vi "SE5082_Create_arb_waveform.vi"(5 "Reference phase (deg)":dbl, 7 "Reference frequency (MHz)":dbl=500.0, 8 "Variables":T1=[{"Value"=10.0, "Variable"="dummy", "Save with Image"=FALSE}, {"Value"=-0.0001, "Variable"="HI", "Save with Image"=FALSE}, {"Value"=-0.0002, "Variable"="LO", "Save with Image"=FALSE}, {"Value"=0.0, "Variable"="dummy1", "Save with Image"=FALSE}, {"Value"=0.0, "Variable"="dummy2", "Save with Image"=FALSE}, {"Value"=0.0, "Variable"="dummy3", "Save with Image"=FALSE}, {"Value"=0.0, "Variable"="tLEDuv", "Save with Image"=FALSE}, {"Value"=1000.0, "Variable"="tMOT0", "Save with Image"=FALSE}, {"Value"=20.0, "Variable"="tMOT1", "Save with Image"=FALSE}, {"Value"=40.0, "Variable"="tMOT2", "Save with Image"=FALSE}, {"Value"=50.0, "Variable"="tMOT3", "Save with Image"=FALSE}, {"Value"=13.0, "Variable"="tMOT3delayREP", "Save with Image"=FALSE}, {"Value"=0.05, "Variable"="tREP", "Save with Image"=FALSE}, {"Value"=0.75, "Variable"="dMOT0", "Save with Image"=FALSE}, {"Value"=1.75, "Variable"="dMOT1", "Save with Image"=FALSE}, {"Value"=1.75, "Variable"="dMOT2", "Save with Image"=FALSE}, {"Value"=0.0, "Variable"="dummy5", "Save with Image"=FALSE}, {"Value"=1.45, "Variable"="pMOT0", "Save with Image"=FALSE}, {"Value"=1.45, "Variable"="pMOT1", "Save with Image"=FALSE}, {"Value"=1.25, "Variable"="pMOT2", "Save with Image"=FALSE}, {"Value"=-1.0, "Variable"="dummy6", "Save with Image"=FALSE}, {"Value"=1.6, "Variable"="pRP0", "Save with Image"=FALSE}, {"Value"=1.6, "Variable"="pRP1", "Save with Image"=FALSE}, {"Value"=0.8, "Variable"="pRP2", "Save with Image"=FALSE}, {"Value"=0.0, "Variable"="MOTdummy0", "Save with Image"=FALSE}, {"Value"=-1.0, "Variable"="MOTdummy1", "Save with Image"=FALSE}, {"Value"=0.0, "Variable"="MOTdummy2", "Save with Image"=FALSE}, {"Value"=0.0, "Variable"="MOTdummy3", "Save with Image"=FALSE}, {"Value"=0.0, "Variable"="MOTdummy4", "Save with Image"=FALSE}, {"Value"=1.8, "Variable"="pCROSS0", "Save with Image"=FALSE}, {"Value"=1.29, "Variable"="pCROSS1", "Save with Image"=FALSE}, {"Value"=1.05, "Variable"="pCROSS2", "Save with Image"=FALSE}, {"Value"=0.75, "Variable"="pCROSS3", "Save with Image"=FALSE}, {"Value"=0.0, "Variable"="pCROSS4", "Save with Image"=FALSE}, {"Value"=5.0, "Variable"="pDIMPL0", "Save with Image"=FALSE}, {"Value"=4.4, "Variable"="pDIMPL1", "Save with Image"=FALSE}, {"Value"=3.65, "Variable"="pDIMPL2", "Save with Image"=FALSE}, {"Value"=3.55, "Variable"="pDIMPL3", "Save with Image"=FALSE}, {"Value"=3.45, "Variable"="pDIMPL4", "Save with Image"=FALSE}, {"Value"=1.8, "Variable"="pTightTrap", "Save with Image"=FALSE}, {"Value"=400.0, "Variable"="tHOLD", "Save with Image"=FALSE}, {"Value"=740.0, "Variable"="tEVAP1", "Save with Image"=FALSE}, {"Value"=2900.0, "Variable"="tEVAP2", "Save with Image"=FALSE}, {"Value"=590.0, "Variable"="tEVAP3", "Save with Image"=FALSE}, {"Value"=50.0, "Variable"="tEVAP4", "Save with Image"=FALSE}, {"Value"=50.0, "Variable"="tHOLDTight", "Save with Image"=FALSE}, {"Value"=0.0, "Variable"="ODTdummy1", "Save with Image"=FALSE}, {"Value"=0.0, "Variable"="ODTdummy2", "Save with Image"=FALSE}, {"Value"=0.0, "Variable"="ODTdummy3", "Save with Image"=FALSE}, {"Value"=0.0, "Variable"="ODTdummy4", "Save with Image"=FALSE}, {"Value"=0.0, "Variable"="ODTdummy5", "Save with Image"=FALSE}, {"Value"=3.59, "Variable"="dIMGx", "Save with Image"=FALSE}, {"Value"=3.59, "Variable"="dIMGx0", "Save with Image"=FALSE}, {"Value"=1.38, "Variable"="dIMGz", "Save with Image"=FALSE}, {"Value"=1.98, "Variable"="dEXCz", "Save with Image"=FALSE}, {"Value"=3.0, "Variable"="pABSx", "Save with Image"=FALSE}, {"Value"=1.35, "Variable"="pABSz", "Save with Image"=FALSE}, {"Value"=0.55, "Variable"="pEXCz", "Save with Image"=FALSE}, {"Value"=0.0, "Variable"="TOF", "Save with Image"=FALSE}, {"Value"=10.0, "Variable"="TOFatomFall", "Save with Image"=FALSE}, {"Value"=0.012, "Variable"="tEXP", "Save with Image"=FALSE}, {"Value"=0.2, "Variable"="tEXP2", "Save with Image"=FALSE}, {"Value"=0.082, "Variable"="tEXC", "Save with Image"=FALSE}, {"Value"=0.001, "Variable"="tWaitIoniz", "Save with Image"=FALSE}, {"Value"=0.065, "Variable"="tCAM", "Save with Image"=FALSE}, {"Value"=200.0, "Variable"="tCAMguppy", "Save with Image"=FALSE}, {"Value"=50.0, "Variable"="tCAMreadout", "Save with Image"=FALSE}, {"Value"=-0.002, "Variable"="tTrigDelay", "Save with Image"=FALSE}, {"Value"=0.0, "Variable"="tTrans", "Save with Image"=FALSE}, {"Value"=1.0, "Variable"="tEXCres", "Save with Image"=FALSE}, {"Value"=0.004, "Variable"="tPUMP", "Save with Image"=FALSE}, {"Value"=2.0, "Variable"="pBLUEswitch", "Save with Image"=FALSE}, {"Value"=2.0, "Variable"="pBLUEswitchEIT", "Save with Image"=FALSE}, {"Value"=3.5, "Variable"="dBLUE", "Save with Image"=FALSE}, {"Value"=3.5, "Variable"="dBLUE0", "Save with Image"=FALSE}, {"Value"=1.7, "Variable"="dBLUEdec", "Save with Image"=FALSE}, {"Value"=2.5, "Variable"="dBLUEdec0", "Save with Image"=FALSE}, {"Value"=3.2, "Variable"="dIMPnew", "Save with Image"=FALSE}, {"Value"=1.0, "Variable"="blueON1", "Save with Image"=FALSE}, {"Value"=0.0, "Variable"="blueON2", "Save with Image"=FALSE}, {"Value"=1.0, "Variable"="blueEXCON1", "Save with Image"=FALSE}, {"Value"=0.0, "Variable"="blueEXCON2", "Save with Image"=FALSE}, {"Value"=35.637858, "Variable"="dRydMW", "Save with Image"=FALSE}, {"Value"=16.0, "Variable"="pRydMW", "Save with Image"=FALSE}, {"Value"=50.0, "Variable"="MWduration", "Save with Image"=FALSE}, {"Value"=4.33, "Variable"="bmw0", "Save with Image"=FALSE}, {"Value"=0.02, "Variable"="bmw1", "Save with Image"=FALSE}, {"Value"=0.0, "Variable"="MWdummy1", "Save with Image"=FALSE}, {"Value"=0.0, "Variable"="MWdummy2", "Save with Image"=FALSE}, {"Value"=0.0, "Variable"="MWdummy3", "Save with Image"=FALSE}, {"Value"=4.3, "Variable"="foffset", "Save with Image"=FALSE}, {"Value"=8.64, "Variable"="fdx", "Save with Image"=FALSE}, {"Value"=-5.78, "Variable"="fdy", "Save with Image"=FALSE}, {"Value"=4.0, "Variable"="fdz", "Save with Image"=FALSE}, {"Value"=300.0, "Variable"="CH203", "Save with Image"=FALSE}, {"Value"=160.0, "Variable"="CH215", "Save with Image"=FALSE}, {"Value"=4.0, "Variable"="CH302", "Save with Image"=FALSE}, {"Value"=280.0, "Variable"="CH315", "Save with Image"=FALSE}, {"Value"=0.0, "Variable"="CH202", "Save with Image"=FALSE}, {"Value"=0.0, "Variable"="CH308", "Save with Image"=FALSE}, {"Value"=0.0, "Variable"="EFIELDdummy2", "Save with Image"=FALSE}, {"Value"=0.0, "Variable"="EFIELDdummy3", "Save with Image"=FALSE}, {"Value"=0.0, "Variable"="EFIELDdummy4", "Save with Image"=FALSE}, {"Value"=0.0, "Variable"="EFIELDdummy5", "Save with Image"=FALSE}, {"Value"=0.0, "Variable"="EFIELDdummy6", "Save with Image"=FALSE}, {"Value"=0.0, "Variable"="EFIELDdummy7", "Save with Image"=FALSE}, {"Value"=1.25, "Variable"="bMOT0", "Save with Image"=FALSE}, {"Value"=2.5, "Variable"="bMOT1", "Save with Image"=FALSE}, {"Value"=2.5, "Variable"="bMOT2", "Save with Image"=FALSE}, {"Value"=1.25, "Variable"="bMOT3", "Save with Image"=FALSE}, {"Value"=0.0, "Variable"="bCOMPx", "Save with Image"=FALSE}, {"Value"=1.35, "Variable"="bCOMPy", "Save with Image"=FALSE}, {"Value"=0.27, "Variable"="bCOMPz", "Save with Image"=FALSE}, {"Value"=0.7, "Variable"="bCOMPx1", "Save with Image"=FALSE}, {"Value"=1.1, "Variable"="bCOMPy1", "Save with Image"=FALSE}, {"Value"=0.5, "Variable"="bCOMPz1", "Save with Image"=FALSE}, {"Value"=4.35, "Variable"="bxfinal", "Save with Image"=FALSE}, {"Value"=0.0, "Variable"="byfinal", "Save with Image"=FALSE}, {"Value"=0.0, "Variable"="bzfinal", "Save with Image"=FALSE}, {"Value"=0.0, "Variable"="BFIELDdummy1", "Save with Image"=FALSE}, {"Value"=0.0, "Variable"="BFIELDdummy2", "Save with Image"=FALSE}, {"Value"=0.0, "Variable"="BFIELDdummy3", "Save with Image"=FALSE}, {"Value"=10.0, "Variable"="tCOILsettle", "Save with Image"=FALSE}, {"Value"=0.0, "Variable"="tRemove", "Save with Image"=FALSE}, {"Value"=3.6, "Variable"="pRemove", "Save with Image"=FALSE}, {"Value"=3.1, "Variable"="dF2CLEAN1x", "Save with Image"=FALSE}, {"Value"=20.0, "Variable"="tF2CLEAN1x", "Save with Image"=FALSE}, {"Value"=4.0, "Variable"="tF2CLEAN2x", "Save with Image"=FALSE}, {"Value"=0.0, "Variable"="tDelayDown", "Save with Image"=FALSE}, {"Value"=156.0, "Variable"="oDDSbluePro", "Save with Image"=FALSE}, {"Value"=-10.25, "Variable"="dDDSbluePro", "Save with Image"=FALSE}, {"Value"=50.0, "Variable"="tRampDDSbluePro", "Save with Image"=FALSE}, {"Value"=416.6261, "Variable"="oDDSred", "Save with Image"=FALSE}, {"Value"=-50.25, "Variable"="dDDSred", "Save with Image"=FALSE}, {"Value"=90.0, "Variable"="tRampDDSred", "Save with Image"=FALSE}, {"Value"=154.0, "Variable"="oDDSblueOld", "Save with Image"=FALSE}, {"Value"=10.0, "Variable"="dDDSblueOld", "Save with Image"=FALSE}, {"Value"=100.0, "Variable"="tRampDDSblueOld", "Save with Image"=FALSE}, {"Value"=1.0, "Variable"="mwON", "Save with Image"=FALSE}, {"Value"=9.4e-05, "Variable"="tRabi", "Save with Image"=FALSE}, {"Value"=9.4e-05, "Variable"="tRabi2", "Save with Image"=FALSE}, {"Value"=5e-05, "Variable"="tRamsey", "Save with Image"=FALSE}, {"Value"=0.0, "Variable"="tRamsey2", "Save with Image"=FALSE}, {"Value"=0.0, "Variable"="tDDSa", "Save with Image"=FALSE}, {"Value"=0.0, "Variable"="tDDSb", "Save with Image"=FALSE}, {"Value"=399.942, "Variable"="dDDSa", "Save with Image"=FALSE}, {"Value"=399.942, "Variable"="dDDSa2", "Save with Image"=FALSE}, {"Value"=0.2, "Variable"="pDDSa", "Save with Image"=FALSE}, {"Value"=1e-07, "Variable"="pDDSa2", "Save with Image"=FALSE}, {"Value"=0.0, "Variable"="phiDDSa", "Save with Image"=FALSE}, {"Value"=0.875, "Variable"="phiDDSa2", "Save with Image"=FALSE}, {"Value"=399.942, "Variable"="dDDSb", "Save with Image"=FALSE}, {"Value"=400.009, "Variable"="dDDSb2", "Save with Image"=FALSE}, {"Value"=0.25, "Variable"="pDDSb", "Save with Image"=FALSE}, {"Value"=1e-07, "Variable"="pDDSb2", "Save with Image"=FALSE}, {"Value"=0.25, "Variable"="phiDDSb", "Save with Image"=FALSE}, {"Value"=0.55, "Variable"="phiDDSb2", "Save with Image"=FALSE}, {"Value"=300.0, "Variable"="tDipole", "Save with Image"=FALSE}, {"Value"=0.7, "Variable"="bCOMPx2", "Save with Image"=FALSE}, {"Value"=0.8, "Variable"="bCOMPy2", "Save with Image"=FALSE}, {"Value"=0.6, "Variable"="bCOMPz2", "Save with Image"=FALSE}, {"Value"=20.0, "Variable"="dMOTRamp1", "Save with Image"=FALSE}, {"Value"=18.0, "Variable"="DMOTload", "Save with Image"=FALSE}, {"Value"=50.0, "Variable"="dMOTRamp2", "Save with Image"=FALSE}, {"Value"=272.0, "Variable"="DMOTimag", "Save with Image"=FALSE}, {"Value"=1000.0, "Variable"="oDDShyperfine", "Save with Image"=FALSE}, {"Value"=0.1, "Variable"="dDDShyperfine", "Save with Image"=FALSE}, {"Value"=0.0, "Variable"="tof", "Save with Image"=FALSE}, {"Value"=262.5, "Variable"="dOPump", "Save with Image"=FALSE}, {"Value"=4500.0, "Variable"="tRampOPump", "Save with Image"=FALSE}, {"Value"=10.0, "Variable"="tOPump", "Save with Image"=FALSE}, {"Value"=1.5, "Variable"="bCOMPx3", "Save with Image"=FALSE}, {"Value"=0.8, "Variable"="bCOMPy3", "Save with Image"=FALSE}, {"Value"=0.0, "Variable"="bCOMPz3", "Save with Image"=FALSE}, {"Value"=0.0, "Variable"="bCOMPx4", "Save with Image"=FALSE}, {"Value"=0.0, "Variable"="bCOMPy4", "Save with Image"=FALSE}, {"Value"=0.0, "Variable"="bCOMPz4", "Save with Image"=FALSE}, {"Value"=0.0, "Variable"="scan2photRes", "Save with Image"=FALSE}, {"Value"=0.0, "Variable"="tEXCsmallProbe", "Save with Image"=FALSE}, {"Value"=0.082, "Variable"="tEXCBlue", "Save with Image"=FALSE}, {"Value"=0.0015, "Variable"="tDownPump", "Save with Image"=FALSE}, {"Value"=98.75, "Variable"="RF1freq1", "Save with Image"=FALSE}, {"Value"=0.1, "Variable"="RF1freq2", "Save with Image"=FALSE}, {"Value"=98.75, "Variable"="dummya", "Save with Image"=FALSE}, {"Value"=0.011, "Variable"="dummyb", "Save with Image"=FALSE}] {"Value" format="%#.9g"}, 10 "waveform sequence":T3=[{"Waveform name"="Init X", "sequence duration (us)"=0.0, "Waveform"=[{"Segment number"=0, "frequency"="500", "phase"="0", "amplitude"="1", "duration"="dummyb", "envelope"=0}]}, {"Waveform name"="WAHUHA", "sequence duration (us)"=0.0, "Waveform"=[{"Segment number"=0, "frequency"="500", "phase"="0", "amplitude"="1", "duration"="0.01", "envelope"=0}, {"Segment number"=0, "frequency"="500", "phase"="0", "amplitude"="0", "duration"="0.01", "envelope"=0}, {"Segment number"=0, "frequency"="500", "phase"="90", "amplitude"="1", "duration"="0.01", "envelope"=0}, {"Segment number"=0, "frequency"="500", "phase"="90", "amplitude"="0", "duration"="0.02", "envelope"=0}, {"Segment number"=0, "frequency"="500", "phase"="270", "amplitude"="1", "duration"="0.01", "envelope"=0}, {"Segment number"=0, "frequency"="500", "phase"="270", "amplitude"="0", "duration"="0.01", "envelope"=0}, {"Segment number"=0, "frequency"="500", "phase"="180", "amplitude"="1", "duration"="0.01", "envelope"=0}, {"Segment number"=0, "frequency"="500", "phase"="180", "amplitude"="0", "duration"="0.01", "envelope"=0}]}, {"Waveform name"="Readout", "sequence duration (us)"=0.0, "Waveform"=[{"Segment number"=0, "frequency"="500", "phase"="0", "amplitude"="1", "duration"="0.03", "envelope"=0}]}] {"Waveform"."envelope" items=["Square", "Gaussian"]}, 11 "AWG sequence_variables":T2={"Sampling rate"=5000000000, "Channel"=1, "Sequence name"=0, "Save sequence"=FALSE, "Load waveform"=FALSE, "Waveform"=[{"Sequence on"=TRUE, "segment name"=0, "repeat"="1", "delay time"="0.001"}, {"Sequence on"=TRUE, "segment name"=1, "repeat"="1", "delay time"="0.005"}, {"Sequence on"=TRUE, "segment name"=2, "repeat"="1", "delay time"="0"}]} {"Sequence name" items=["Init X", "WAHUHA", "Readout X", "New waveform..."]; "Channel" format="%.0p"; "Sampling rate" format="%.0p"; "Waveform"."segment name" items=["Init X", "WAHUHA", "Readout X"]}) -> (1 "ref amplitude":dbl[](array[numeric]), 2 "y":dbl[](array[numeric]), 3 "x":dbl[](array[numeric]))   [LabVIEW 2017]
uses:
  waveform_variables_new.ctl
  sequence_variables.ctl
  Software/Rydberg_Control/TypeDefinition/variables.ctl
panel:
  out "size ref (new)":i32=4736
  out "size ref":i32=4736
  out "size y (new)":i32=4736
  out "segment name":string[](array[string])
  out "Step size (ns)":dbl=0.2
  out "XY Graph all":cluster{dbl[], "y":dbl[]}[](graph)
  out "XY Graph":cluster{dbl[], "y":dbl[]}[](graph)
  out "all duration":i32[](array[numeric])=[55, 50, 50, 50, 100, 50, 50, 50, 50, 50, 50, 50, 100, 50, 50, 50, 50, 50, 50, 50, 100, 50, 50, 50, 50, 50, 50, 50, 100, 50, 50, 50, 50, 50, 50, 50, 100, 50, 50, 50, 50, 50, 50, 50, 100, 50, 50, 50, 50, 50, 50, 50, 100, 50, 50, 50, 50, 50, 50, 50, 100, 50, 50, 50, 50, 50, 50, 50, 100, 50, 50, 50, 50, 50, 50, 50, 100, 50, 50, 50, 50, 150, 30]
  out "all frequency":dbl[](array[numeric])=[500.0, 500.0, 500.0, 500.0, 500.0, 500.0, 500.0, 500.0, 500.0, 500.0, 500.0, 500.0, 500.0, 500.0, 500.0, 500.0, 500.0, 500.0, 500.0, 500.0, 500.0, 500.0, 500.0, 500.0, 500.0, 500.0, 500.0, 500.0, 500.0, 500.0, 500.0, 500.0, 500.0, 500.0, 500.0, 500.0, 500.0, 500.0, 500.0, 500.0, 500.0, 500.0, 500.0, 500.0, 500.0, 500.0, 500.0, 500.0, 500.0, 500.0, 500.0, 500.0, 500.0, 500.0, 500.0, 500.0, 500.0, 500.0, 500.0, 500.0, 500.0, 500.0, 500.0, 500.0, 500.0, 500.0, 500.0, 500.0, 500.0, 500.0, 500.0, 500.0, 500.0, 500.0, 500.0, 500.0, 500.0, 500.0, 500.0, 500.0, 500.0, 500.0, 500.0]
  out "all phase":dbl[](array[numeric])=[0.0, 0.0, 0.0, 90.0, 90.0, 270.0, 270.0, 180.0, 180.0, 0.0, 0.0, 90.0, 90.0, 270.0, 270.0, 180.0, 180.0, 0.0, 0.0, 90.0, 90.0, 270.0, 270.0, 180.0, 180.0, 0.0, 0.0, 90.0, 90.0, 270.0, 270.0, 180.0, 180.0, 0.0, 0.0, 90.0, 90.0, 270.0, 270.0, 180.0, 180.0, 0.0, 0.0, 90.0, 90.0, 270.0, 270.0, 180.0, 180.0, 0.0, 0.0, 90.0, 90.0, 270.0, 270.0, 180.0, 180.0, 0.0, 0.0, 90.0, 90.0, 270.0, 270.0, 180.0, 180.0, 0.0, 0.0, 90.0, 90.0, 270.0, 270.0, 180.0, 180.0, 0.0, 0.0, 90.0, 90.0, 270.0, 270.0, 180.0, 180.0, 0.0, 0.0]
  out "all amplitude":dbl[](array[numeric])=[1.0, 1.0, 0.0, 1.0, 0.0, 1.0, 0.0, 1.0, 0.0, 1.0, 0.0, 1.0, 0.0, 1.0, 0.0, 1.0, 0.0, 1.0, 0.0, 1.0, 0.0, 1.0, 0.0, 1.0, 0.0, 1.0, 0.0, 1.0, 0.0, 1.0, 0.0, 1.0, 0.0, 1.0, 0.0, 1.0, 0.0, 1.0, 0.0, 1.0, 0.0, 1.0, 0.0, 1.0, 0.0, 1.0, 0.0, 1.0, 0.0, 1.0, 0.0, 1.0, 0.0, 1.0, 0.0, 1.0, 0.0, 1.0, 0.0, 1.0, 0.0, 1.0, 0.0, 1.0, 0.0, 1.0, 0.0, 1.0, 0.0, 1.0, 0.0, 1.0, 0.0, 1.0, 0.0, 1.0, 0.0, 1.0, 0.0, 1.0, 0.0, 1.0, 0.0]
  out "time for waveform":dbl[](array[numeric])=[0.0, 1.1e-08, 2.1e-08, 3.1e-08, 4.1e-08, 6.1e-08, 7.1e-08, 8.1e-08, 9.1e-08, 1.01e-07, 1.11e-07, 1.21e-07, 1.31e-07, 1.51e-07, 1.61e-07, 1.71e-07, 1.81e-07, 1.91e-07, 2.01e-07, 2.11e-07, 2.21e-07, 2.41e-07, 2.51e-07, 2.61e-07, 2.71e-07, 2.81e-07, 2.91e-07, 3.01e-07, 3.11e-07, 3.31e-07, 3.41e-07, 3.51e-07, 3.61e-07, 3.71e-07, 3.81e-07, 3.91e-07, 4.01e-07, 4.21e-07, 4.31e-07, 4.41e-07, 4.51e-07, 4.61e-07, 4.71e-07, 4.81e-07, 4.91e-07, 5.11e-07, 5.21e-07, 5.31e-07, 5.41e-07, 5.51e-07, 5.61e-07, 5.71e-07, 5.81e-07, 6.01e-07, 6.11e-07, 6.21e-07, 6.31e-07, 6.41e-07, 6.51e-07, 6.61e-07, 6.71e-07, 6.91e-07, 7.01e-07, 7.11e-07, 7.21e-07, 7.31e-07, 7.41e-07, 7.51e-07, 7.61e-07, 7.81e-07, 7.91e-07, 8.01e-07, 8.11e-07, 8.21e-07, 8.31e-07, 8.41e-07, 8.51e-07, 8.71e-07, 8.81e-07, 8.91e-07, 9.01e-07, 9.11e-07, 9.41e-07]
  out "input amplitude":dbl[](array[numeric])=[1.0, 1.0, 0.0, 1.0, 0.0, 1.0, 0.0, 1.0, 0.0, 1.0, 0.0, 1.0, 0.0, 1.0, 0.0, 1.0, 0.0, 1.0, 0.0, 1.0, 0.0, 1.0, 0.0, 1.0, 0.0, 1.0, 0.0, 1.0, 0.0, 1.0, 0.0, 1.0, 0.0, 1.0, 0.0, 1.0, 0.0, 1.0, 0.0, 1.0, 0.0, 1.0, 0.0, 1.0, 0.0, 1.0, 0.0, 1.0, 0.0, 1.0, 0.0, 1.0, 0.0, 1.0, 0.0, 1.0, 0.0, 1.0, 0.0, 1.0, 0.0, 1.0, 0.0, 1.0, 0.0, 1.0, 0.0, 1.0, 0.0, 1.0, 0.0, 1.0, 0.0, 1.0, 0.0, 1.0, 0.0, 1.0, 0.0, 1.0, 0.0, 1.0]
  out "input phase":dbl[](array[numeric])=[0.0, 0.0, 0.0, 90.0, 90.0, 270.0, 270.0, 180.0, 180.0, 0.0, 0.0, 90.0, 90.0, 270.0, 270.0, 180.0, 180.0, 0.0, 0.0, 90.0, 90.0, 270.0, 270.0, 180.0, 180.0, 0.0, 0.0, 90.0, 90.0, 270.0, 270.0, 180.0, 180.0, 0.0, 0.0, 90.0, 90.0, 270.0, 270.0, 180.0, 180.0, 0.0, 0.0, 90.0, 90.0, 270.0, 270.0, 180.0, 180.0, 0.0, 0.0, 90.0, 90.0, 270.0, 270.0, 180.0, 180.0, 0.0, 0.0, 90.0, 90.0, 270.0, 270.0, 180.0, 180.0, 0.0, 0.0, 90.0, 90.0, 270.0, 270.0, 180.0, 180.0, 0.0, 0.0, 90.0, 90.0, 270.0, 270.0, 180.0, 180.0, 0.0]
  out "input frequency":dbl[](array[numeric])=[500.0, 500.0, 500.0, 500.0, 500.0, 500.0, 500.0, 500.0, 500.0, 500.0, 500.0, 500.0, 500.0, 500.0, 500.0, 500.0, 500.0, 500.0, 500.0, 500.0, 500.0, 500.0, 500.0, 500.0, 500.0, 500.0, 500.0, 500.0, 500.0, 500.0, 500.0, 500.0, 500.0, 500.0, 500.0, 500.0, 500.0, 500.0, 500.0, 500.0, 500.0, 500.0, 500.0, 500.0, 500.0, 500.0, 500.0, 500.0, 500.0, 500.0, 500.0, 500.0, 500.0, 500.0, 500.0, 500.0, 500.0, 500.0, 500.0, 500.0, 500.0, 500.0, 500.0, 500.0, 500.0, 500.0, 500.0, 500.0, 500.0, 500.0, 500.0, 500.0, 500.0, 500.0, 500.0, 500.0, 500.0, 500.0, 500.0, 500.0, 500.0, 500.0]
  out "input duration":i32[](array[numeric])=[55, 50, 50, 50, 100, 50, 50, 50, 50, 50, 50, 50, 100, 50, 50, 50, 50, 50, 50, 50, 100, 50, 50, 50, 50, 50, 50, 50, 100, 50, 50, 50, 50, 50, 50, 50, 100, 50, 50, 50, 50, 50, 50, 50, 100, 50, 50, 50, 50, 50, 50, 50, 100, 50, 50, 50, 50, 50, 50, 50, 100, 50, 50, 50, 50, 50, 50, 50, 100, 50, 50, 50, 50, 50, 50, 50, 100, 50, 50, 50, 50, 150]
  out "repeat":i32[](array[numeric])=[1, 10, 1]
  out "segment number":u16[](array[numeric])=[0, 1, 2]
  out "sequence on":bool[](array[boolean])=[TRUE, TRUE, TRUE]
  in  "Plot waveform":bool
  in  "Waveform name":u16(ring) items=["Init X", "WAHUHA", "Readout X", "New waveform..."]
  in  "Save waveform":bool
  out "size y":i32=4736
  out "total samples":i32=4736
  out "samples to add":i32=30
  out "segment init phase":dbl[](array[numeric])=[0.0, 179.99999999999977, 180.00000000000045, 180.0, 180.00000000000182, 179.99999999999818, 180.0, 180.0, 180.0, 180.0, 180.0, 180.00000000000364, 180.0, 180.0, 179.99999999999636, 180.0, 180.0, 180.0, 180.0, 180.0, 180.0, 180.00000000000728, 180.00000000000728, 180.00000000000728, 179.99999999999272, 179.99999999999272, 179.99999999999272, 180.0, 180.0, 180.0, 180.00000000000728, 180.0, 180.00000000000728, 180.0, 180.0, 180.0, 180.0, 180.00000000001455, 180.0, 180.0, 180.0, 180.0, 180.0, 180.00000000001455, 180.0, 180.0, 180.00000000001455, 180.0, 180.0, 180.00000000001455, 180.0, 180.00000000001455, 180.0, 180.0000000000291, 180.0, 179.99999999998545, 179.99999999998545, 180.0, 179.99999999998545, 180.0, 180.00000000001455, 180.0, 180.00000000001455, 179.99999999998545, 180.0, 180.0, 180.0, 179.9999999999709, 180.0, 180.0, 180.0000000000291, 180.0, 180.0, 180.0, 180.0, 180.0, 180.0000000000291, 180.0, 180.0, 180.0, 180.0000000000291, 180.0000000000291, 180.0]
  out "ref phase(deg)":dbl[](array[numeric])
  out "Reference phase":cluster{"x":dbl[], "y":dbl[]}(graph)
  out "Plot X":dbl[](graph)
  out "Plot Y":dbl[](graph)
  out "y (original)":dbl[](array[numeric])
  out "Sampling rate":i64=5000000000
  out "Reference amplitude":cluster{"x":dbl[], "y":dbl[]}(graph)
  # "Max 5 GSa/s"
  # "1 or 2"
  # "ON?"
  # "segment name"
  # "repeat"
  # "delay time (us)"
  # "No."
  # "freq (MHz)"
  # "phase  (deg)"
  # "amplitude (0-1)"
  # "duration (us)"
  # "envelope"
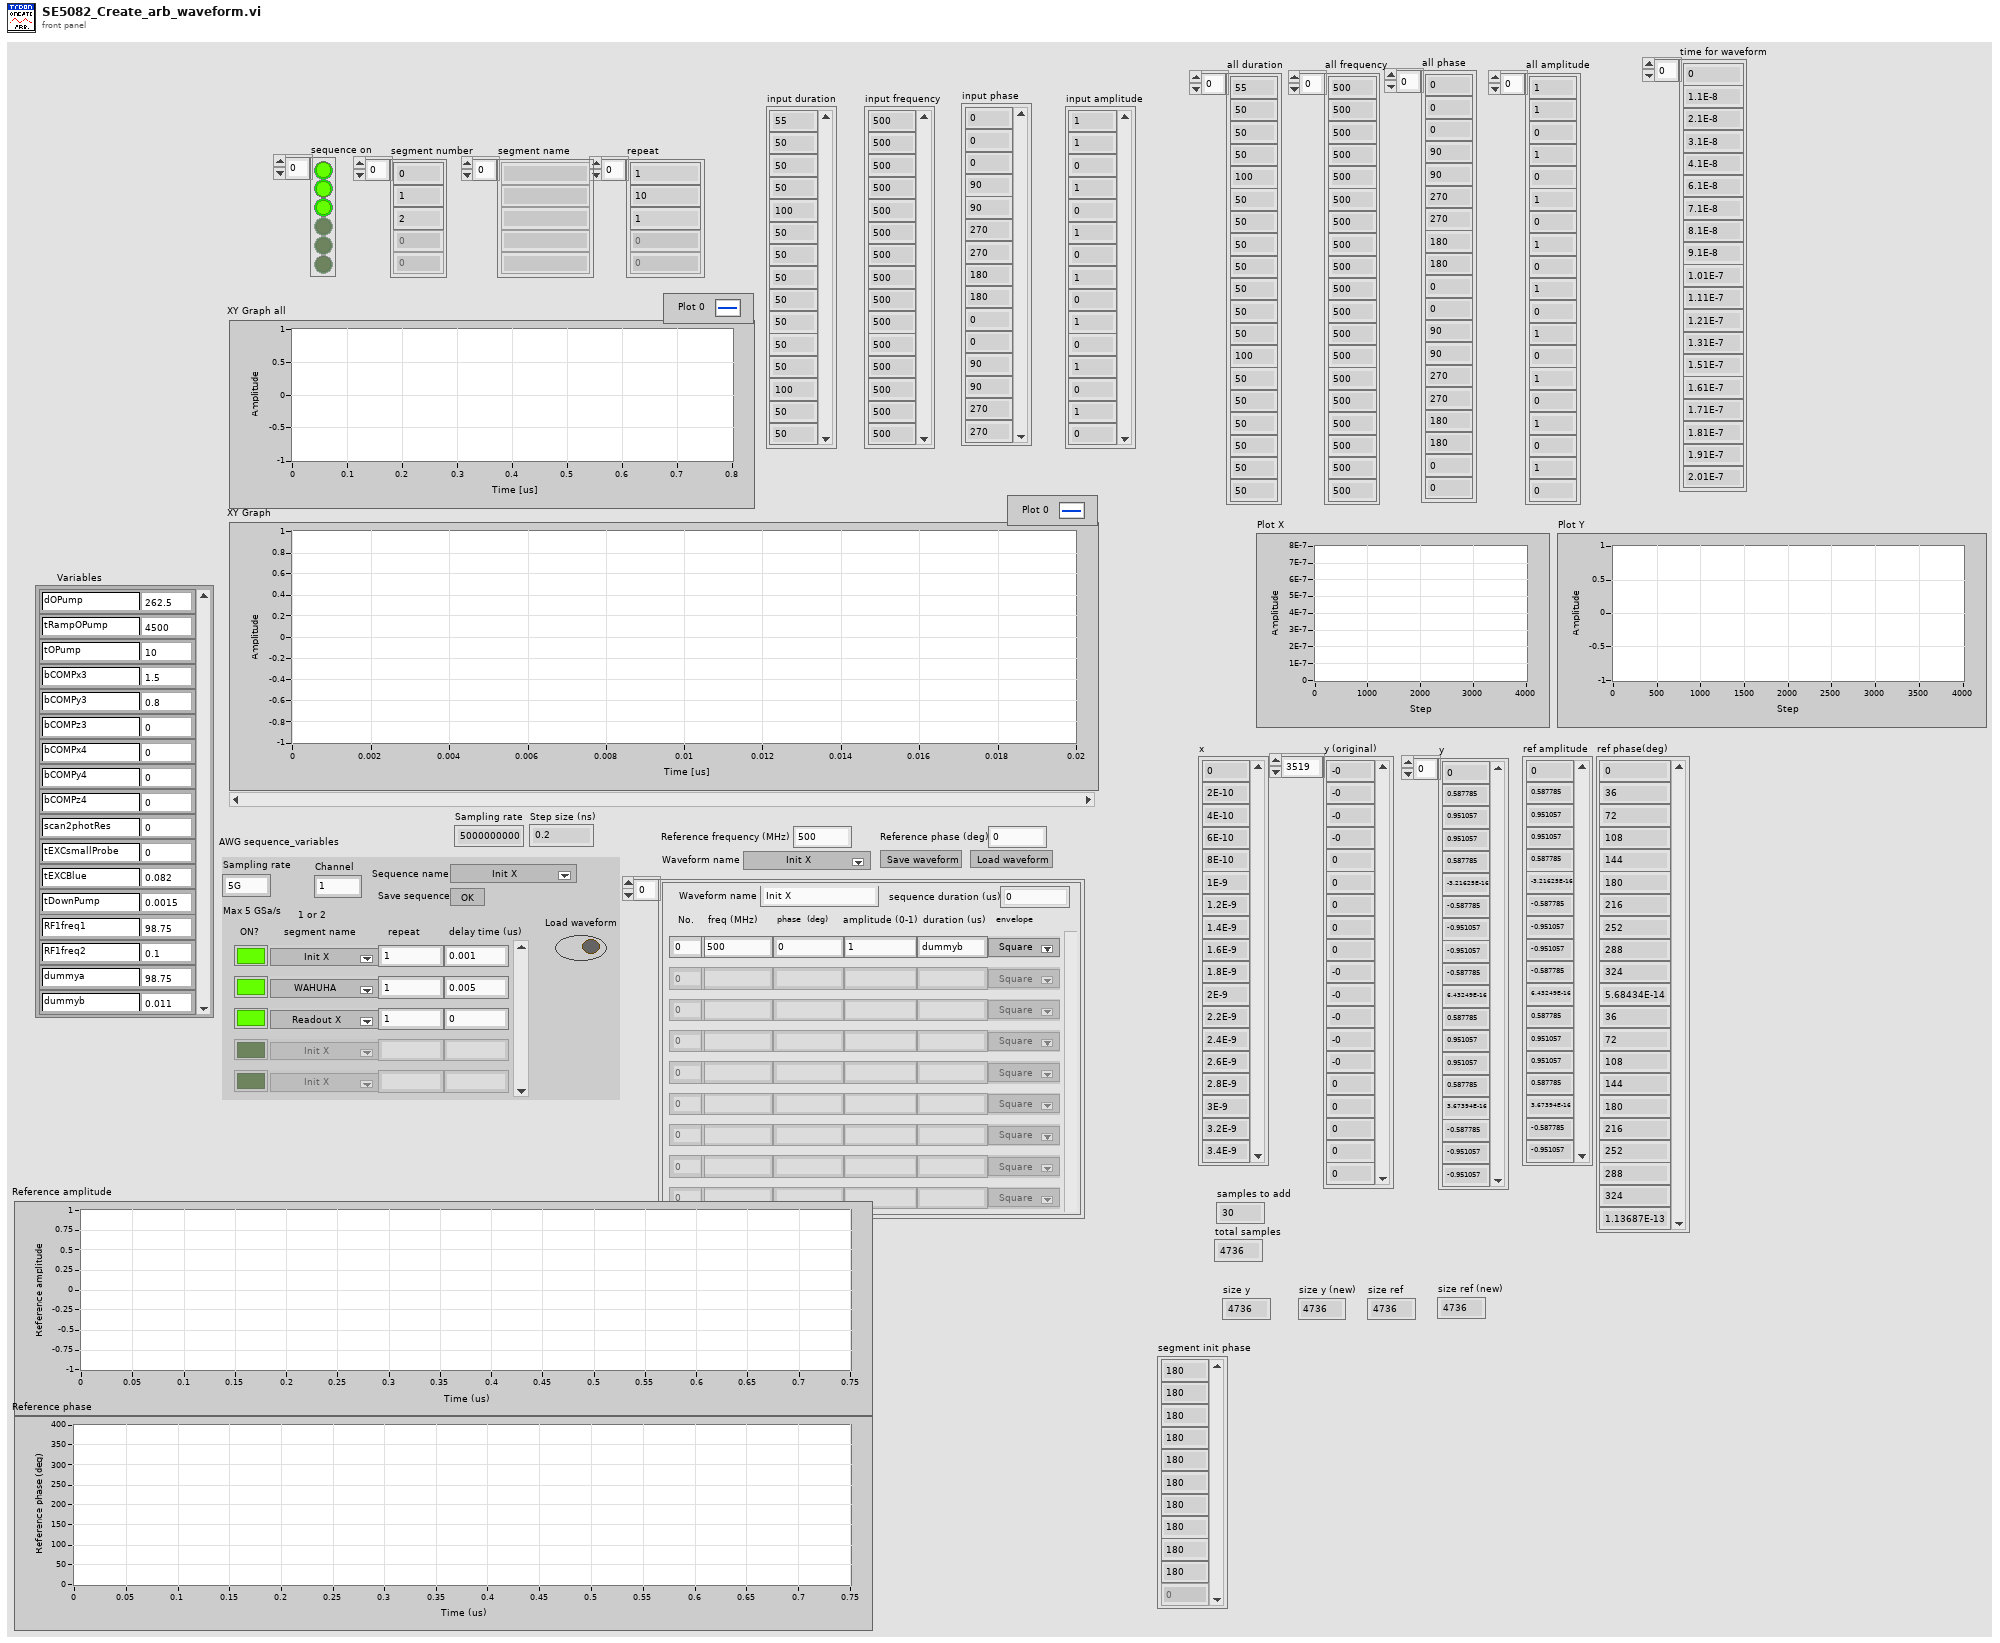
[diagram p1: front panel]
types:
  T1 = typedef "variables.ctl" = cluster{"Value":dbl, "Variable":string, "Save with Image":bool}[]
  T2 = typedef "sequence_variables.ctl" = cluster{"Sampling rate":i64, "Channel":i8, "Sequence name":u16, "Save sequence":bool, "Load waveform":bool, "Waveform":cluster{"Sequence on":bool, "segment name":u16, "repeat":string, "delay time":string}[]}
  T3 = typedef "waveform_variables_new.ctl" = cluster{"Waveform name":string, "sequence duration (us)":dbl, "Waveform":cluster{"Segment number":i32, "frequency":string, "phase":string, "amplitude":string, "duration":string, "envelope":u16}[]}[]
  T4 = cluster{"Sequence on":bool, "segment name":u16, "repeat":string, "delay time":string}[]
  T5 = cluster{"Waveform name":string, "sequence duration (us)":dbl, "Waveform":cluster{"Segment number":i32, "frequency":string, "phase":string, "amplitude":string, "duration":string, "envelope":u16}[]}
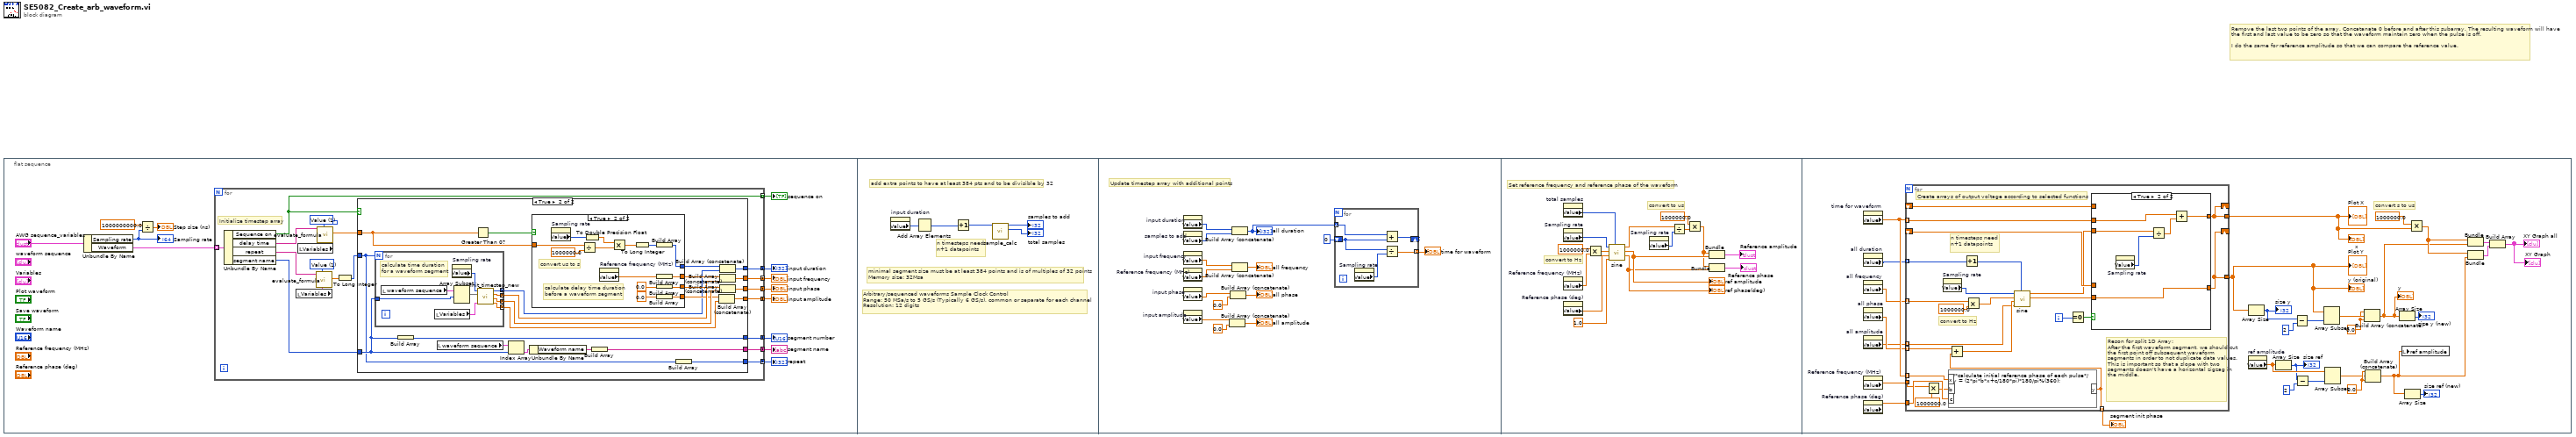
[diagram p0: block diagram]
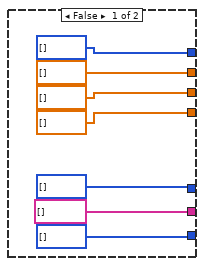
[diagram p2: hidden frame]
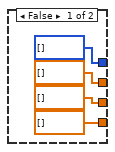
[diagram p3: hidden frame]
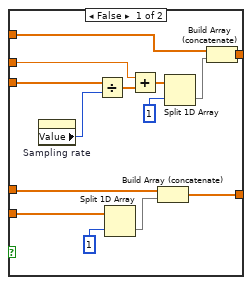
[diagram p4: hidden frame]
diagram:
  # "Remove the last two points of the array. Concatanate 0 before and after this subarray. The resulting waveform will have the first and last value to be zero so that the waveform maintain zero when the pulse is off.\n\nI do the same for reference amplitude so that we can compare the reference value."
  n1 = flat-sequence {
    frame #0 {
      n2 = Unbundle By Name("AWG sequence_variables") -> ("Sampling rate"=w10:i64, "Waveform"=w5:T4)
      "Sampling rate" <- w10
      n3 = Divide(x=1000000000.0, y=w10) -> (x/y=→"Step size (ns)":dbl)
      n4 = for {
        tunnel: w5 -> [w32] mode=indexing
        tunnel: [w26] -> w3 mode=indexing
        tunnel: [w18] -> w4 mode=concatenating
        tunnel: [w24] -> w9 mode=concatenating
        tunnel: [w23] -> w6 mode=concatenating
        tunnel: [w22] -> w7 mode=concatenating
        tunnel: [w21] -> w8 mode=concatenating
        tunnel: [w20] -> w12 mode=concatenating
        tunnel: [w19] -> w13 mode=concatenating
        w14 = u16 1 items=["Time in counts", "Value"] ("Time or Value")
        w30 = u16 1 items=["Time in counts", "Value"] ("Time or Value")
        # "Initialize timestep array"
        n5 = Unbundle By Name(w32) -> ("Sequence on"=w26:bool, "delay time"=w27:string, "repeat"=w16:string, "segment name"=w15:u16)
        n6 = local read "Variables"() -> (w31:T1)
        n7 = local read "Variables"() -> (w28:T1)
        n8 = call "evaluate_formula.vi"("Variable array"=w31, "Time or Value"=w30, "Formula"=w16) -> ("Output"=w29:dbl)  [unwired: 7 in, 1 out]
        n9 = call "evaluate_formula.vi"("Variable array"=w28, "Time or Value"=w14, "Formula"=w27) -> ("Output"=w17:dbl)  [unwired: 7 in, 1 out]
        n10 = To Long Integer(number=w29) -> (32bit integer=w25:i32)
        n11 = case shown="True" w26 {
          tunnel: w15 -> [_ w56]
          tunnel: w25 -> [_ w55]
          tunnel: [i32[] [] ("segment duration (int)") w51] -> w24
          tunnel: [dbl[] [] ("segment frequency") w49] -> w23
          tunnel: [dbl[] [] ("segment phase") w48] -> w22
          tunnel: [dbl[] [] ("segment amplitude") w47] -> w21
          tunnel: [string[] [] w58] -> w20
          tunnel: [u16[] [] w57] -> w19
          tunnel: [i32[] [] w54] -> w18
          tunnel: w17 -> [_ w52]
          frame False {
          }
          frame True {
            n12 = for {
              N: w55 -> [_]
              tunnel: w56 -> [w84]
              tunnel: [w83] -> w40 mode=concatenating
              tunnel: [w82] -> w46 mode=concatenating
              tunnel: [w81] -> w45 mode=concatenating
              tunnel: [w80] -> w44 mode=concatenating
              # "calculate time duration\nfor a waveform segment"
              n13 = local read "waveform sequence"() -> (w87:T3)
              n14 = local read "Variables"() -> (w85:T1)
              n15 = property on="Sampling rate" class="DigNum (strict)"() -> ("Value"=w86:i64)  [unwired: 2 in, 2 out]
              n16 = Array Subset(array=w87, index=w84) -> (w88:T3)  [unwired: 1 in]
              n17 = call "Init_timestep_new.vi"("Variables"=w85, "waveform sequence"=w88, "Sampling rate"=w86) -> ("segment amplitude"=w80:dbl[], "segment phase"=w81:dbl[], "segment frequency"=w82:dbl[], "segment duration (int)"=w83:i32[])  [unwired: 5 in]
            }
            n18 = Build Array(w56) -> (w57:u16[])
            n19 = local read "waveform sequence"() -> (w61:T3)
            n20 = Greater Than 0?(x=w52) -> (x > 0?=w53:bool)
            n21 = Index Array(array=w61, index=w56) -> (element=w60:T5)
            n22 = Unbundle By Name(w60) -> ("Waveform name"=w59:string)
            n23 = case shown="True" w53 {
              tunnel: w52 -> [_ w76]
              tunnel: [i32[] [] w74] -> w50
              tunnel: [dbl[] [] w70] -> w43
              tunnel: [dbl[] [] w69] -> w42
              tunnel: [dbl[] [] w68] -> w41
              frame False {
              }
              frame True {
                # "calculate delay time duration\nbefore a waveform segment"
                # "convert us to s"
                n24 = property on="Sampling rate" class="DigNum (strict)"() -> ("Value"=w67:i64)  [unwired: 2 in, 2 out]
                n25 = Divide(x=w76, y=1000000.0) -> (x/y=w78:dbl)
                n26 = To Double Precision Float(number=w67) -> (double precision float=w66:dbl)
                n27 = property on="Reference frequency (MHz)" class="DigNum (strict)"() -> ("Value"=w73:dbl)  [unwired: 2 in, 2 out]
                n28 = Multiply(x=w66, y=w78) -> (x*y=w79:dbl)
                n29 = To Long Integer(number=w79) -> (32bit integer=w75:i32)
                n30 = Build Array(w75) -> (w74:i32[])
                n31 = Build Array(w73) -> (w70:dbl[])
                n32 = Build Array(0.0 ("element")) -> (w69:dbl[])
                n33 = Build Array(0.0 ("element")) -> (w68:dbl[])
              }
            }
            n34 = Build Array(w59) -> (w58:string[])
            n35 = Build Array(w55) -> (w54:i32[])
            n36 = Build Array (concatenate)(w41, w44) -> (w47:dbl[])
            n37 = Build Array (concatenate)(w50, w40) -> (w51:i32[])
            n38 = Build Array (concatenate)(w43, w46) -> (w49:dbl[])
            n39 = Build Array (concatenate)(w42, w45) -> (w48:dbl[])
          }
        }
      }
      "sequence on" <- w3
      "segment number" <- w13
      "repeat" <- w4
      "input duration" <- w9
      "input frequency" <- w6
      "input phase" <- w7
      "input amplitude" <- w8
      "segment name" <- w12
    }
    frame #1 {
      # "minimal segment size must be at least 384 points and is of multiples of 32 points\nMemory size: 32Msa"
      # "Arbitrary/sequenced waveforms Sample Clock Control\nRange: 50 MSa/s to 5 GS/s (Typically 6 GS/s), common or separate for each channel\nResolution: 12 digits"
      # "n timesteps need n+1 datapoints"
      # "add extra points to have at least 384 pts and to be divisible by 32"
      n40 = property on="input duration" class="Arr (strict)"() -> ("Value"=w89:i32[])  [unwired: 2 in, 2 out]
      n41 = Add Array Elements(numeric array=w89) -> (sum=w91:i32)
      n42 = Increment(x=w91) -> (x+1=w90:i32)
      n43 = call "sample_calc.vi"("Input samples"=w90) -> ("total samples"=→"total samples":i32, "samples to add"=→"samples to add":i32)  [unwired: 9 in]
    }
    frame #2 {
      # "Update timestep array with additional points"
      n44 = property on="input duration" class="Arr (strict)"() -> ("Value"=w107:i32[])  [unwired: 2 in, 2 out]
      n45 = property on="samples to add" class="DigNum (strict)"() -> ("Value"=w106:i32)  [unwired: 2 in, 2 out]
      n46 = property on="input frequency" class="Arr (strict)"() -> ("Value"=w102:dbl[])  [unwired: 2 in, 2 out]
      n47 = property on="Reference frequency (MHz)" class="DigNum (strict)"() -> ("Value"=w97:dbl)  [unwired: 2 in, 2 out]
      n48 = property on="input phase" class="Arr (strict)"() -> ("Value"=w101:dbl[])  [unwired: 2 in, 2 out]
      n49 = property on="input amplitude" class="Arr (strict)"() -> ("Value"=w100:dbl[])  [unwired: 2 in, 2 out]
      n50 = Build Array (concatenate)(w100, 0.0) -> (→"all amplitude":dbl[])
      n51 = Build Array (concatenate)(w101, 0.0) -> (→"all phase":dbl[])
      n52 = Build Array (concatenate)(w107, w106) -> (w94:i32[])
      "all duration" <- w94
      n53 = Build Array (concatenate)(w102, w97) -> (→"all frequency":dbl[])
      n54 = for {
        tunnel: w94 -> [w111] mode=indexing
        shift-right: [w110] -> _
        shift-left: 0 -> [w109]
        tunnel: [w108] -> w96 mode=indexing
        n55 = property on="Sampling rate" class="DigNum (strict)"() -> ("Value"=w112:i64)  [unwired: 2 in, 2 out]
        n56 = Add(x=w111, y=w109) -> (x+y=w110:i32)
        n57 = Divide(x=w109, y=w112) -> (x/y=w108:dbl)
      }
      "time for waveform" <- w96
    }
    frame #3 {
      # "convert to us"
      # "convert to Hz"
      # "Set reference frequency and reference phase of the waveform"
      n58 = property on="total samples" class="DigNum (strict)"() -> ("Value"=w121:i32)  [unwired: 2 in, 2 out]
      n59 = property on="Sampling rate" class="DigNum (strict)"() -> ("Value"=w122:i64)  [unwired: 2 in, 2 out]
      n60 = property on="Reference frequency (MHz)" class="DigNum (strict)"() -> ("Value"=w114:dbl)  [unwired: 2 in, 2 out]
      n61 = property on="Reference phase (deg)" class="DigNum (strict)"() -> ("Value"=w113:dbl)  [unwired: 2 in, 2 out]
      n62 = Multiply(x=1000000.0 ("y"), y=w114) -> (x*y=w127:dbl)
      n63 = call "sine.vi"("number of x points"=w121, "amplitude"=1.0, "phase"=w113, "frequency"=w127, "Sampling rate"=w122) -> ("phase out (deg)"=w124:dbl[], "y"=w128:dbl[], "x"=w117:dbl[])  [unwired: 4 in]
      "ref phase(deg)" <- w124
      "ref amplitude" <- w128
      n64 = property on="Sampling rate" class="DigNum (strict)"() -> ("Value"=w116:i64)  [unwired: 2 in, 2 out]
      n65 = Divide(x=w117, y=w116) -> (x/y=w119:dbl[])
      n66 = Multiply(x=1000000.0 ("y"), y=w119) -> (x*y=w115:dbl[])
      n67 = Bundle(w115, "y"=w128) -> (→"Reference amplitude":cluster{dbl[], "y":dbl[]})  [unwired: 1 in]
      n68 = Bundle(w115, "phase out (deg)"=w124) -> (→"Reference phase":cluster{dbl[], "phase out (deg)":dbl[]})  [unwired: 1 in]
    }
    frame #4 {
      w134 = 0.0 ("element")
      w139 = 0.0 ("element")
      # "convert s to us"
      n69 = property on="time for waveform" class="Arr (strict)"() -> ("Value"=w157:dbl[])  [unwired: 2 in, 2 out]
      n70 = property on="all duration" class="Arr (strict)"() -> ("Value"=w154:i32[])  [unwired: 2 in, 2 out]
      n71 = property on="all frequency" class="Arr (strict)"() -> ("Value"=w153:dbl[])  [unwired: 2 in, 2 out]
      n72 = property on="all phase" class="Arr (strict)"() -> ("Value"=w152:dbl[])  [unwired: 2 in, 2 out]
      n73 = property on="all amplitude" class="Arr (strict)"() -> ("Value"=w151:dbl[])  [unwired: 2 in, 2 out]
      n74 = property on="Reference frequency (MHz)" class="DigNum (strict)"() -> ("Value"=w155:dbl)  [unwired: 2 in, 2 out]
      n75 = property on="Reference phase (deg)" class="DigNum (strict)"() -> ("Value"=w156:dbl)  [unwired: 2 in, 2 out]
      n76 = for {
        tunnel: w154 -> [w163] mode=indexing
        shift-right: [w179] -> _
        shift-left: _ -> [w180]
        tunnel: [w179] -> w144
        shift-right: [w176] -> _
        shift-left: _ -> [w177]
        tunnel: [w176] -> w150
        tunnel: w157 -> [w175] mode=indexing
        tunnel: w157 -> [w171] mode=indexing
        tunnel: w155 -> [w166]
        tunnel: w156 -> [w169]
        tunnel: [w164] -> w158 mode=indexing
        tunnel: w153 -> [w161] mode=indexing
        tunnel: w152 -> [w160] mode=indexing
        tunnel: w151 -> [w159] mode=indexing
        i -> [w181]
        # "n timesteps need n+1 datapoints"
        # "convert to Hz"
        # "Create arrays of output voltage according to selected functions"
        # "Reson for split 1D Array:\nAfter the first waveform segment, we should cut the first point off subsequent waveform segments in order to not duplicate data values. This is important so that a slope with two segments doesn't have a horizontal zigzag in the middle."
        n77 = Multiply(x=w166, y=1000000.0) -> (x*y=w165:dbl)
        n78 = property on="Sampling rate" class="DigNum (strict)"() -> ("Value"=w168:i64)  [unwired: 2 in, 2 out]
        n79 = formula code="/*calculate initial reference phase of each pulse*/\ny = (2*pi*b*x+c/180*pi)*180/pi%(360);"("x"=w171, "b"=w165, "c"=w169) -> ("y"=w164:dbl)
        n80 = Add(x=w160, y=w164) -> (x+y=w170:dbl)
        n81 = Increment(x=w163) -> (x+1=w162:i32)
        n82 = Multiply(x=w161, y=1000000.0) -> (x*y=w172:dbl)
        n83 = call "sine.vi"("number of x points"=w162, "amplitude"=w159, "phase"=w170, "frequency"=w172, "Sampling rate"=w168) -> ("y"=w182:dbl[], "x"=w178:dbl[])  [unwired: 4 in, 1 out]
        n84 = Equal To 0?(x=w181) -> (x = 0?=w174:bool)
        n85 = case shown="True" w174 {
          tunnel: w182 -> [w189 w202]
          tunnel: [w193 w202] -> w179
          tunnel: w180 -> [w194 _]
          tunnel: w178 -> [w185 w201]
          tunnel: [w191 w198] -> w176
          tunnel: w177 -> [w192 _]
          tunnel: w175 -> [w186 w200]
          frame False {
            n86 = property on="Sampling rate" class="DigNum (strict)"() -> ("Value"=w183:i64)  [unwired: 2 in, 2 out]
            n87 = Divide(x=w185, y=w183) -> (x/y=w187:dbl[])
            n88 = Split 1D Array(array=w189, index=1) -> (second subarray=w188:dbl[])  [unwired: 1 out]
            n89 = Add(x=w186, y=w187) -> (x+y=w184:dbl[])
            n90 = Build Array (concatenate)(w194, w188) -> (w193:dbl[])
            n91 = Split 1D Array(array=w184, index=1) -> (second subarray=w190:dbl[])  [unwired: 1 out]
            n92 = Build Array (concatenate)(w192, w190) -> (w191:dbl[])
          }
          frame True {
            n93 = property on="Sampling rate" class="DigNum (strict)"() -> ("Value"=w197:i64)  [unwired: 2 in, 2 out]
            n94 = Divide(x=w201, y=w197) -> (x/y=w199:dbl[])
            n95 = Add(x=w200, y=w199) -> (x+y=w198:dbl[])
          }
        }
      }
      "y (original)" <- w144
      "x" <- w150
      "Plot Y" <- w144
      "Plot X" <- w150
      "segment init phase" <- w158
      n96 = Array Size(array=w144) -> (size(s)=w141:i32)
      "size y" <- w141
      n97 = property on="ref amplitude" class="Arr (strict)"() -> ("Value"=w132:dbl[])  [unwired: 2 in, 2 out]
      n98 = Array Size(array=w132) -> (size(s)=w131:i32)
      "size ref" <- w131
      n99 = Subtract(x=w141, y=2) -> (x-y=w142:i32)
      n100 = Subtract(x=w131, y=2) -> (x-y=w135:i32)
      n101 = Array Subset(array=w144, length=w142) -> (w143:dbl[])  [unwired: 1 in]
      n102 = Array Subset(array=w132, length=w135) -> (w133:dbl[])  [unwired: 1 in]
      n103 = Build Array (concatenate)(w139, w143, w139) -> (w137:dbl[])
      "y" <- w137
      n104 = Build Array (concatenate)(w134, w133, w134) -> (w129:dbl[])
      n105 = Array Size(array=w137) -> (size(s)=→"size y (new)":i32)
      n106 = local write "ref amplitude"(w129) -> ()
      n107 = Array Size(array=w129) -> (size(s)=→"size ref (new)":i32)
      n108 = Multiply(x=1000000.0 ("y"), y=w150) -> (x*y=w148:dbl[])
      n109 = Bundle(w148, w137) -> (w147:cluster{dbl[], dbl[]})  [unwired: 1 in]
      n110 = Bundle(w148, w129) -> (w146:cluster{dbl[], dbl[]})  [unwired: 1 in]
      n111 = Build Array(w147, w146) -> (→"XY Graph" →"XY Graph all":cluster{dbl[], dbl[]}[])
    }
  }
